vi "benchmark-DataContainer.vi"() -> (2 "read":dbl=1.454608345031738e-06 format="%#_6f", 3 "write":dbl=7.281229972839357e-07 format="%#_6f")   [LabVIEW 2017]
uses:
  0f9e4dc8-5c94-49e2-bb31-afcfc0247ef6.vi
  f88afbd5-defc-4e1d-9497-5b20b3cf386f.vi
  Data Container Folder/Support/Unflatten DataCNT to DVR.vi
  Data Container Folder/Data Container.lvlib
  <userlib>/_OpenG.lib/md5/md5.llb/MD5 Message Digest (Binary String)__ogtk.vi
panel:
  out "length":i32=1170
  out "outside":i32=499
  out "unit (ms)":cluster{dbl[]}[](graph)=[{[1.5038490295410156e-06, 1.503896713256836e-06, 1.4037609100341798e-06, 1.5039443969726562e-06, 1.503896713256836e-06, 1.4055252075195312e-06, 1.5020847320556641e-06, 1.5039920806884766e-06, 1.4037132263183594e-06, 1.503896713256836e-06, 1.4036178588867187e-06, 1.5039920806884766e-06, 1.503896713256836e-06, 1.4037132263183594e-06, 1.503896713256836e-06, 1.5039443969726562e-06, 1.4036655426025392e-06, 1.5039443969726562e-06, 1.4036655426025392e-06, 1.503896713256836e-06, 1.5039443969726562e-06, 1.40380859375e-06, 1.5038490295410156e-06, 1.4037132263183594e-06, 1.503896713256836e-06, 1.5039920806884766e-06, 1.4037132263183594e-06, 1.503896713256836e-06, 1.4036655426025392e-06, 1.4036178588867187e-06, 1.503896713256836e-06, 1.4037132263183594e-06, 1.503896713256836e-06, 1.4038562774658204e-06, 1.503753662109375e-06, 1.4036655426025392e-06, 1.4037609100341798e-06, 1.5039443969726562e-06, 1.503896713256836e-06, 1.5039443969726562e-06, 1.4036655426025392e-06, 1.5038490295410156e-06, 1.5039920806884766e-06, 1.5039443969726562e-06, 1.4037609100341798e-06, 1.503896713256836e-06, 1.5039443969726562e-06, 1.4036655426025392e-06, 1.503896713256836e-06, 1.6042709350585937e-06, 1.4035701751708983e-06, 1.4037132263183594e-06, 1.5039920806884766e-06, 1.503896713256836e-06, 1.4037132263183594e-06, 1.503896713256836e-06, 1.4036655426025392e-06, 1.4037132263183594e-06, 1.503896713256836e-06, 1.4036655426025392e-06, 1.5039443969726562e-06, 1.4036655426025392e-06, 1.4037132263183594e-06, 1.503896713256836e-06, 1.4036655426025392e-06, 1.5038490295410156e-06, 1.4037609100341798e-06, 1.4037609100341798e-06, 1.503896713256836e-06, 1.4036655426025392e-06, 1.5039443969726562e-06, 1.4036655426025392e-06, 1.5039920806884766e-06, 1.4036178588867187e-06, 1.4037609100341798e-06, 1.503896713256836e-06, 1.4036178588867187e-06, 1.4037609100341798e-06, 1.5039443969726562e-06, 1.4036655426025392e-06, 1.5039920806884766e-06, 1.4036178588867187e-06, 1.503896713256836e-06, 1.4036655426025392e-06, 1.4037132263183594e-06, 1.4036655426025392e-06, 1.5039443969726562e-06, 1.4035701751708983e-06, 1.5040874481201172e-06, 1.5039443969726562e-06, 1.4036655426025392e-06, 1.503896713256836e-06, 1.4037132263183594e-06, 1.503896713256836e-06, 1.4037132263183594e-06, 1.4035701751708983e-06, 1.5039920806884766e-06, 1.4037132263183594e-06, 1.503896713256836e-06, 1.4036655426025392e-06, 1.4037132263183594e-06, 1.503896713256836e-06, 1.4037132263183594e-06, 1.503896713256836e-06, 1.4036655426025392e-06, 1.4037132263183594e-06, 1.503896713256836e-06, 1.4036655426025392e-06, 1.5039443969726562e-06, 1.4036655426025392e-06, 1.4037132263183594e-06, 1.503896713256836e-06, 1.4036655426025392e-06, 1.604175567626953e-06, 1.4037609100341798e-06, 1.503896713256836e-06, 1.4037132263183594e-06, 1.5038490295410156e-06, 1.4037609100341798e-06, 1.5039920806884766e-06, 1.4035701751708983e-06, 1.4037132263183594e-06, 1.503896713256836e-06, 1.4036655426025392e-06, 1.5040397644042968e-06, 1.4035701751708983e-06, 1.4037132263183594e-06, 1.503896713256836e-06, 1.4036655426025392e-06, 1.4037132263183594e-06, 1.503896713256836e-06, 1.4036655426025392e-06, 1.4037132263183594e-06, 1.503896713256836e-06, 1.4036655426025392e-06, 1.4037132263183594e-06, 1.503896713256836e-06, 1.5039920806884766e-06, 1.4036178588867187e-06, 1.6042232513427735e-06, 1.5039443969726562e-06, 1.4036655426025392e-06, 1.4041900634765624e-06, 1.5034198760986327e-06, 1.4036655426025392e-06, 1.5039443969726562e-06, 1.4036655426025392e-06, 1.5039443969726562e-06, 1.4036655426025392e-06, 1.4036655426025392e-06, 1.8048286437988282e-06, 1.804637908935547e-06, 1.503896713256836e-06, 1.5039443969726562e-06, 1.5039920806884766e-06, 1.4036655426025392e-06, 1.5039443969726562e-06, 1.5039920806884766e-06, 1.4035701751708983e-06, 1.5039443969726562e-06, 1.4036655426025392e-06, 1.5039443969726562e-06, 1.4036655426025392e-06, 1.503896713256836e-06, 1.4037609100341798e-06, 1.5039443969726562e-06, 1.4036655426025392e-06, 1.5039443969726562e-06, 1.4035701751708983e-06, 1.4037132263183594e-06, 1.5039920806884766e-06, 1.4036655426025392e-06, 1.5039443969726562e-06, 1.4036655426025392e-06, 1.503896713256836e-06, 1.4037132263183594e-06, 1.503896713256836e-06, 1.4036655426025392e-06, 1.4037132263183594e-06, 1.503896713256836e-06, 1.4037132263183594e-06, 1.503896713256836e-06, 1.4036655426025392e-06, 1.5040397644042968e-06, 1.5038013458251954e-06, 1.4037132263183594e-06, 1.4036655426025392e-06, 1.5039920806884766e-06, 1.4036655426025392e-06, 1.4037132263183594e-06, 1.503896713256836e-06, 1.4037132263183594e-06, 1.503896713256836e-06, 1.4036655426025392e-06, 1.4037132263183594e-06, 1.503896713256836e-06, 1.4036655426025392e-06, 1.5039443969726562e-06, 1.4036655426025392e-06, 1.5039443969726562e-06, 1.4036655426025392e-06, 1.503896713256836e-06, 1.4037132263183594e-06, 1.503896713256836e-06, 1.4037609100341798e-06, 1.5038490295410156e-06, 1.4036655426025392e-06, 1.5040397644042968e-06, 1.4036655426025392e-06, 1.5038490295410156e-06, 1.4037609100341798e-06, 1.503896713256836e-06, 1.4036655426025392e-06, 1.5039443969726562e-06, 1.4036178588867187e-06, 1.4037132263183594e-06, 1.5039443969726562e-06, 1.4036655426025392e-06, 1.5039443969726562e-06, 1.503896713256836e-06, 1.4037132263183594e-06, 1.5039920806884766e-06, 1.4035701751708983e-06, 1.4037132263183594e-06, 1.5039920806884766e-06, 1.503896713256836e-06, 1.4036178588867187e-06, 1.5039920806884766e-06, 1.4036655426025392e-06, 1.5039443969726562e-06, 1.4036655426025392e-06, 1.4037132263183594e-06, 1.503896713256836e-06, 1.4036655426025392e-06, 1.5039443969726562e-06, 1.4036655426025392e-06, 1.5039443969726562e-06, 1.4036655426025392e-06, 1.503896713256836e-06, 1.4037132263183594e-06, 1.503896713256836e-06, 1.4036655426025392e-06, 1.5039443969726562e-06, 1.5039920806884766e-06, 1.4036655426025392e-06, 1.5038490295410156e-06, 1.4037609100341798e-06, 1.5039443969726562e-06, 1.4036655426025392e-06, 1.503896713256836e-06, 1.4037132263183594e-06, 1.503896713256836e-06, 1.4037132263183594e-06, 1.503896713256836e-06, 1.4036655426025392e-06, 1.5039443969726562e-06, 1.5039920806884766e-06, 1.4036655426025392e-06, 1.5039443969726562e-06, 1.4035701751708983e-06, 1.5040397644042968e-06, 1.4036655426025392e-06, 1.5038490295410156e-06, 1.4037609100341798e-06, 1.503896713256836e-06, 1.4037132263183594e-06, 1.503896713256836e-06, 1.4036655426025392e-06, 1.5039443969726562e-06, 1.4036655426025392e-06, 1.4036655426025392e-06, 1.5039443969726562e-06, 1.4036655426025392e-06, 1.5039443969726562e-06, 1.4036655426025392e-06, 1.5039920806884766e-06, 1.4036655426025392e-06, 1.5039443969726562e-06, 1.4036655426025392e-06, 1.5039443969726562e-06, 1.4036655426025392e-06, 1.5039443969726562e-06, 1.4036655426025392e-06, 1.4036655426025392e-06, 1.5039443969726562e-06, 1.4036655426025392e-06, 1.503896713256836e-06, 1.4037132263183594e-06, 1.503896713256836e-06, 1.4036655426025392e-06, 1.5039443969726562e-06, 1.4036655426025392e-06, 1.5039443969726562e-06, 1.4036655426025392e-06, 1.5039920806884766e-06, 1.4037132263183594e-06, 1.5038013458251954e-06, 1.4037132263183594e-06, 1.5039920806884766e-06, 1.4036655426025392e-06, 1.5039443969726562e-06, 1.503896713256836e-06, 1.4036655426025392e-06, 1.5039443969726562e-06, 1.4036655426025392e-06, 1.4037132263183594e-06, 1.503896713256836e-06, 1.4036655426025392e-06, 1.5039920806884766e-06, 1.5038490295410156e-06, 1.4037132263183594e-06, 1.4036655426025392e-06, 1.503896713256836e-06, 1.5040397644042968e-06, 1.4036655426025392e-06, 1.4035701751708983e-06, 1.5040397644042968e-06, 1.4036655426025392e-06, 1.503896713256836e-06, 1.5039443969726562e-06, 1.4036655426025392e-06, 1.5039443969726562e-06, 1.4036655426025392e-06, 1.503896713256836e-06, 1.5039443969726562e-06, 1.4037609100341798e-06, 1.503896713256836e-06, 1.5039443969726562e-06, 1.503896713256836e-06, 1.4037132263183594e-06, 1.503896713256836e-06, 1.4037132263183594e-06, 1.4035701751708983e-06, 1.5039920806884766e-06, 1.5039443969726562e-06, 1.4036655426025392e-06, 1.4036655426025392e-06, 1.5039443969726562e-06, 1.4036655426025392e-06, 1.5039443969726562e-06, 1.4036655426025392e-06, 1.5039920806884766e-06, 1.4036655426025392e-06, 1.5039443969726562e-06, 1.4036655426025392e-06, 1.5039443969726562e-06, 1.4036655426025392e-06, 1.5039443969726562e-06, 1.4036655426025392e-06, 1.503896713256836e-06, 1.4037132263183594e-06, 1.4036655426025392e-06, 1.503896713256836e-06, 1.5039443969726562e-06, 1.4037609100341798e-06, 1.503896713256836e-06, 1.4035224914550781e-06, 1.5040874481201172e-06, 1.4036178588867187e-06, 1.5039920806884766e-06, 1.4036178588867187e-06, 1.503896713256836e-06, 1.4041423797607422e-06, 1.5035629272460938e-06, 1.4036655426025392e-06, 1.503896713256836e-06, 1.4037132263183594e-06, 1.503896713256836e-06, 1.4036655426025392e-06, 1.5039443969726562e-06, 1.5039920806884766e-06, 1.4036655426025392e-06, 1.4036178588867187e-06, 1.5039920806884766e-06, 1.4036178588867187e-06, 1.4036655426025392e-06, 1.5039443969726562e-06, 1.4037609100341798e-06, 1.503896713256836e-06, 1.4036655426025392e-06, 1.5039443969726562e-06, 1.503896713256836e-06, 1.4037132263183594e-06, 1.5039920806884766e-06, 1.4035701751708983e-06, 1.5039443969726562e-06, 1.4037609100341798e-06, 1.4036178588867187e-06, 1.503896713256836e-06, 1.4036655426025392e-06, 1.5039443969726562e-06, 1.4036655426025392e-06, 1.5039920806884766e-06, 1.4036178588867187e-06, 1.5039920806884766e-06, 1.4036655426025392e-06, 1.5050411224365234e-06, 1.4025688171386718e-06, 1.604175567626953e-06, 1.4037609100341798e-06, 1.4035701751708983e-06, 1.5039443969726562e-06, 1.4036655426025392e-06, 1.5039443969726562e-06, 1.4036655426025392e-06, 1.5039443969726562e-06, 1.4036655426025392e-06, 1.503896713256836e-06, 1.4037609100341798e-06, 1.4036178588867187e-06, 1.503896713256836e-06, 1.4037132263183594e-06, 1.503896713256836e-06, 1.4037609100341798e-06, 1.5038490295410156e-06, 1.4036655426025392e-06, 1.5039443969726562e-06, 1.40380859375e-06, 1.5038490295410156e-06, 1.4037132263183594e-06, 1.503896713256836e-06, 1.4036655426025392e-06, 1.4037132263183594e-06, 1.503896713256836e-06, 1.4036655426025392e-06, 1.5039443969726562e-06, 1.4036655426025392e-06, 1.5039443969726562e-06, 1.4036655426025392e-06, 1.4036655426025392e-06, 1.5039920806884766e-06, 1.4036178588867187e-06, 1.5039443969726562e-06, 1.4036655426025392e-06, 1.5039920806884766e-06, 1.4036655426025392e-06, 1.4037132263183594e-06, 1.503896713256836e-06, 1.4036178588867187e-06, 1.5039920806884766e-06, 1.4036655426025392e-06, 1.5039443969726562e-06, 1.4036655426025392e-06, 1.4036655426025392e-06, 1.5039443969726562e-06, 1.4036655426025392e-06, 1.5039443969726562e-06, 1.4036655426025392e-06, 1.4036655426025392e-06, 1.5039443969726562e-06, 1.4036655426025392e-06, 1.5039443969726562e-06, 1.4036655426025392e-06, 1.5039920806884766e-06, 1.4036178588867187e-06, 1.4036655426025392e-06, 1.503896713256836e-06, 1.4037132263183594e-06, 1.503896713256836e-06, 1.4037132263183594e-06, 1.4036655426025392e-06, 1.5039920806884766e-06, 1.4036178588867187e-06, 1.5039920806884766e-06, 1.4035701751708983e-06, 1.4037132263183594e-06, 1.5039920806884766e-06, 1.5038490295410156e-06, 1.4037609100341798e-06, 1.503896713256836e-06, 1.4038562774658204e-06, 1.4035224914550781e-06, 1.503896713256836e-06, 1.4037132263183594e-06, 1.503896713256836e-06, 1.4037609100341798e-06, 1.4036178588867187e-06, 1.503896713256836e-06, 1.4036178588867187e-06, 1.5039920806884766e-06, 1.4037609100341798e-06, 1.5038490295410156e-06, 1.4037609100341798e-06, 1.5038013458251954e-06, 1.4037132263183594e-06, 1.503896713256836e-06, 1.5039920806884766e-06, 1.4037132263183594e-06, 1.503896713256836e-06, 1.5039443969726562e-06, 1.503896713256836e-06, 1.4037609100341798e-06, 1.4037132263183594e-06, 1.5038013458251954e-06, 1.4037132263183594e-06, 1.503896713256836e-06, 1.4037609100341798e-06, 1.5039443969726562e-06, 1.4036655426025392e-06, 1.4043331146240235e-06]}, ...(2 in all)]
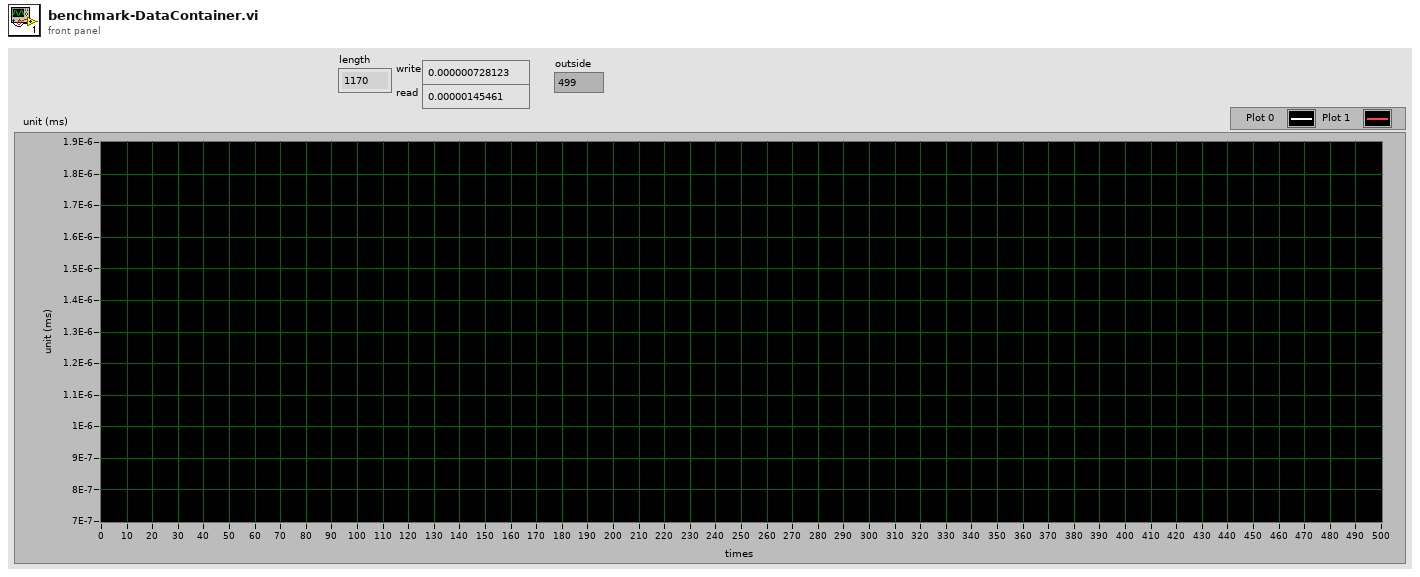
[diagram p1: front panel]
types:
  T1 = cluster{"error constant":errorcluster, "error constant 2":errorcluster, "error constant 3":errorcluster, "error constant 4":errorcluster, "error constant 5":errorcluster, "error constant 6":errorcluster, "error constant 7":errorcluster, "error constant 8":errorcluster, "error constant 9":errorcluster, "error constant 10":errorcluster, "error constant 11":errorcluster, "error constant 12":errorcluster, "error constant 13":errorcluster, "error constant 14":errorcluster, "error constant 15":errorcluster, "error constant 16":errorcluster, "error constant 17":errorcluster, "error constant 18":errorcluster, "error constant 19":errorcluster, "error constant 20":errorcluster, "error constant 21":errorcluster, "error constant 22":errorcluster, "error constant 23":errorcluster, "error constant 24":errorcluster, "error constant 25":errorcluster, "error constant 26":errorcluster, "error constant 27":errorcluster, "error constant 28":errorcluster, "error constant 29":errorcluster, "error constant 30":errorcluster, "error constant 31":errorcluster, "error constant 32":errorcluster, "error constant 33":errorcluster, "error constant 34":errorcluster, "error constant 35":errorcluster, "error constant 36":errorcluster, "error constant 37":errorcluster, "error constant 38":errorcluster, "error constant 39":errorcluster, "error constant 40":errorcluster, "error constant 41":errorcluster, "error constant 42":errorcluster, "error constant 43":errorcluster, "error constant 44":errorcluster, "error constant 45":errorcluster, "error constant 46":errorcluster, "error constant 47":errorcluster, "error constant 48":errorcluster, "error constant 49":errorcluster, "error constant 50":errorcluster, "error constant 51":errorcluster, "error constant 52":errorcluster, "error constant 53":errorcluster, "error constant 54":errorcluster, "error constant 55":errorcluster, "error constant 56":errorcluster, "error constant 57":errorcluster, "error constant 58":errorcluster, "error constant 59":errorcluster, "error constant 60":errorcluster, "error constant 61":errorcluster, "error constant 62":errorcluster, "error constant 63":errorcluster, "error constant 64":errorcluster, "error constant 65":errorcluster, cluster{"error constant":errorcluster, "error constant 2":errorcluster, "error constant 3":errorcluster, "error constant 4":errorcluster, "error constant 5":errorcluster, "error constant 6":errorcluster, "error constant 7":errorcluster, "error constant 8":errorcluster, "error constant 9":errorcluster, "error constant 10":errorcluster, "error constant 11":errorcluster, "error constant 12":errorcluster, "error constant 13":errorcluster, "error constant 14":errorcluster, "error constant 15":errorcluster, "error constant 16":errorcluster, "error constant 17":errorcluster, "error constant 18":errorcluster, "error constant 19":errorcluster, "error constant 20":errorcluster, "error constant 21":errorcluster, "error constant 22":errorcluster, "error constant 23":errorcluster, "error constant 24":errorcluster, "error constant 25":errorcluster, "error constant 26":errorcluster, "error constant 27":errorcluster, "error constant 28":errorcluster, "error constant 29":errorcluster, "error constant 30":errorcluster, "error constant 31":errorcluster, "error constant 32":errorcluster, "error constant 33":errorcluster, "error constant 34":errorcluster, "error constant 35":errorcluster, "error constant 36":errorcluster, "error constant 37":errorcluster, "error constant 38":errorcluster, "error constant 39":errorcluster, "error constant 40":errorcluster, "error constant 41":errorcluster, "error constant 42":errorcluster, "error constant 43":errorcluster, "error constant 44":errorcluster, "error constant 45":errorcluster, "error constant 46":errorcluster, "error constant 47":errorcluster, "error constant 48":errorcluster, "error constant 49":errorcluster, "error constant 50":errorcluster, "error constant 51":errorcluster, "error constant 52":errorcluster, "error constant 53":errorcluster, "error constant 54":errorcluster, "error constant 55":errorcluster, "error constant 56":errorcluster, "error constant 57":errorcluster, "error constant 58":errorcluster, "error constant 59":errorcluster, "error constant 60":errorcluster, "error constant 61":errorcluster, "error constant 62":errorcluster, "error constant 63":errorcluster, "error constant 64":errorcluster, "error constant 65":errorcluster}}
  T2 = typedef "Data Container.lvlib/Def-DataCNT.ctl" = refnum<k1>
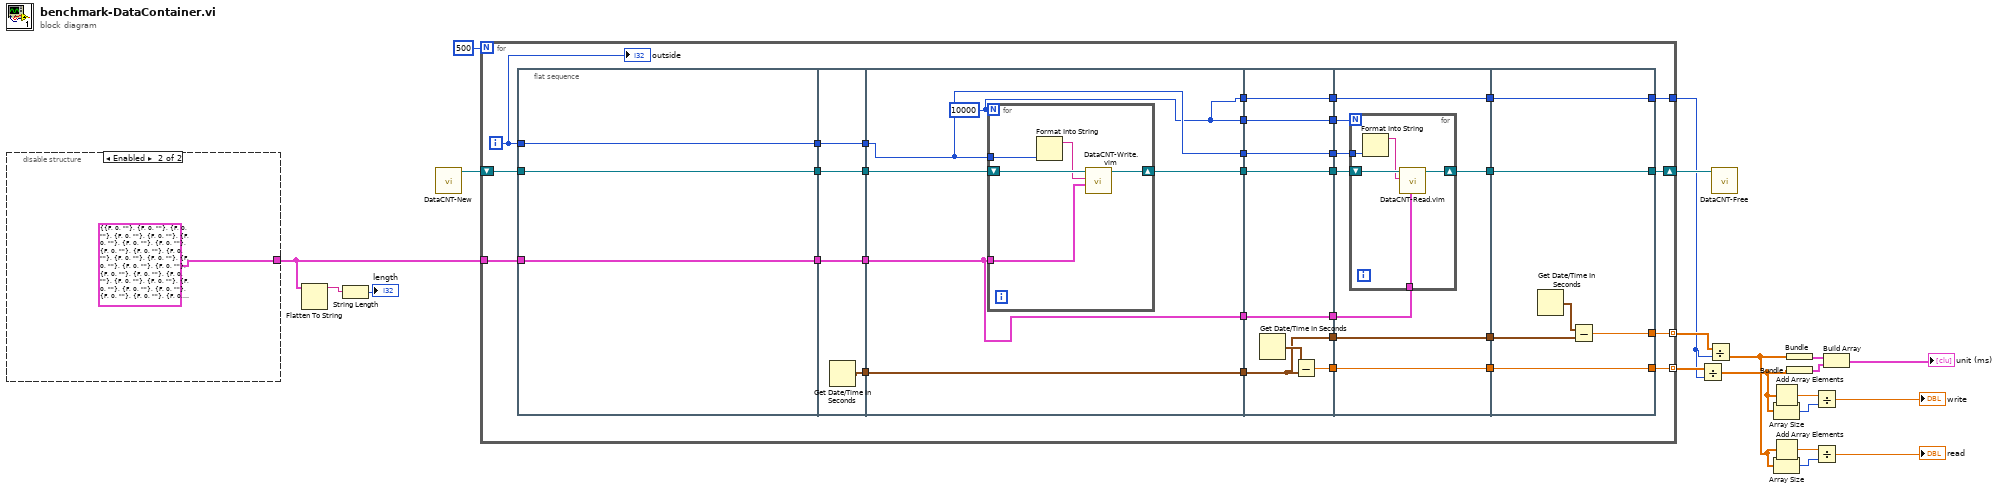
[diagram p0: block diagram]
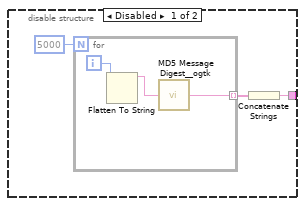
[diagram p2: hidden frame]
diagram:
  n1 = disable-structure shown="Enabled" {
    disable-tunnel: [w21 T1 {"error constant"={"status"=FALSE, "code"=0, "source"=""}, "error constant 2"={"status"=FALSE, "code"=0, "source"=""}, "error constant 3"={"status"=FALSE, "code"=0, "source"=""}, "error constant 4"={"status"=FALSE, "code"=0, "source"=""}, "error constant 5"={"status"=FALSE, "code"=0, "source"=""}, "error constant 6"={"status"=FALSE, "code"=0, "source"=""}, "error constant 7"={"status"=FALSE, "code"=0, "source"=""}, "error constant 8"={"status"=FALSE, "code"=0, "source"=""}, "error constant 9"={"status"=FALSE, "code"=0, "source"=""}, "error constant 10"={"status"=FALSE, "code"=0, "source"=""}, "error constant 11"={"status"=FALSE, "code"=0, "source"=""}, "error constant 12"={"status"=FALSE, "code"=0, "source"=""}, "error constant 13"={"status"=FALSE, "code"=0, "source"=""}, "error constant 14"={"status"=FALSE, "code"=0, "source"=""}, "error constant 15"={"status"=FALSE, "code"=0, "source"=""}, "error constant 16"={"status"=FALSE, "code"=0, "source"=""}, "error constant 17"={"status"=FALSE, "code"=0, "source"=""}, "error constant 18"={"status"=FALSE, "code"=0, "source"=""}, "error constant 19"={"status"=FALSE, "code"=0, "source"=""}, "error constant 20"={"status"=FALSE, "code"=0, "source"=""}, "error constant 21"={"status"=FALSE, "code"=0, "source"=""}, "error constant 22"={"status"=FALSE, "code"=0, "source"=""}, "error constant 23"={"status"=FALSE, "code"=0, "source"=""}, "error constant 24"={"status"=FALSE, "code"=0, "source"=""}, "error constant 25"={"status"=FALSE, "code"=0, "source"=""}, "error constant 26"={"status"=FALSE, "code"=0, "source"=""}, "error constant 27"={"status"=FALSE, "code"=0, "source"=""}, "error constant 28"={"status"=FALSE, "code"=0, "source"=""}, "error constant 29"={"status"=FALSE, "code"=0, "source"=""}, "error constant 30"={"status"=FALSE, "code"=0, "source"=""}, "error constant 31"={"status"=FALSE, "code"=0, "source"=""}, "error constant 32"={"status"=FALSE, "code"=0, "source"=""}, "error constant 33"={"status"=FALSE, "code"=0, "source"=""}, "error constant 34"={"status"=FALSE, "code"=0, "source"=""}, "error constant 35"={"status"=FALSE, "code"=0, "source"=""}, "error constant 36"={"status"=FALSE, "code"=0, "source"=""}, "error constant 37"={"status"=FALSE, "code"=0, "source"=""}, "error constant 38"={"status"=FALSE, "code"=0, "source"=""}, "error constant 39"={"status"=FALSE, "code"=0, "source"=""}, "error constant 40"={"status"=FALSE, "code"=0, "source"=""}, "error constant 41"={"status"=FALSE, "code"=0, "source"=""}, "error constant 42"={"status"=FALSE, "code"=0, "source"=""}, "error constant 43"={"status"=FALSE, "code"=0, "source"=""}, "error constant 44"={"status"=FALSE, "code"=0, "source"=""}, "error constant 45"={"status"=FALSE, "code"=0, "source"=""}, "error constant 46"={"status"=FALSE, "code"=0, "source"=""}, "error constant 47"={"status"=FALSE, "code"=0, "source"=""}, "error constant 48"={"status"=FALSE, "code"=0, "source"=""}, "error constant 49"={"status"=FALSE, "code"=0, "source"=""}, "error constant 50"={"status"=FALSE, "code"=0, "source"=""}, "error constant 51"={"status"=FALSE, "code"=0, "source"=""}, "error constant 52"={"status"=FALSE, "code"=0, "source"=""}, "error constant 53"={"status"=FALSE, "code"=0, "source"=""}, "error constant 54"={"status"=FALSE, "code"=0, "source"=""}, "error constant 55"={"status"=FALSE, "code"=0, "source"=""}, "error constant 56"={"status"=FALSE, "code"=0, "source"=""}, "error constant 57"={"status"=FALSE, "code"=0, "source"=""}, "error constant 58"={"status"=FALSE, "code"=0, "source"=""}, "error constant 59"={"status"=FALSE, "code"=0, "source"=""}, "error constant 60"={"status"=FALSE, "code"=0, "source"=""}, "error constant 61"={"status"=FALSE, "code"=0, "source"=""}, "error constant 62"={"status"=FALSE, "code"=0, "source"=""}, "error constant 63"={"status"=FALSE, "code"=0, "source"=""}, "error constant 64"={"status"=FALSE, "code"=0, "source"=""}, "error constant 65"={"status"=FALSE, "code"=0, "source"=""}, {"error constant"={"status"=FALSE, "code"=0, "source"=""}, "error constant 2"={"status"=FALSE, "code"=0, "source"=""}, "error constant 3"={"status"=FALSE, "code"=0, "source"=""}, "error constant 4"={"status"=FALSE, "code"=0, "source"=""}, "error constant 5"={"status"=FALSE, "code"=0, "source"=""}, "error constant 6"={"status"=FALSE, "code"=0, "source"=""}, "error constant 7"={"status"=FALSE, "code"=0, "source"=""}, "error constant 8"={"status"=FALSE, "code"=0, "source"=""}, "error constant 9"={"status"=FALSE, "code"=0, "source"=""}, "error constant 10"={"status"=FALSE, "code"=0, "source"=""}, "error constant 11"={"status"=FALSE, "code"=0, "source"=""}, "error constant 12"={"status"=FALSE, "code"=0, "source"=""}, "error constant 13"={"status"=FALSE, "code"=0, "source"=""}, "error constant 14"={"status"=FALSE, "code"=0, "source"=""}, "error constant 15"={"status"=FALSE, "code"=0, "source"=""}, "error constant 16"={"status"=FALSE, "code"=0, "source"=""}, "error constant 17"={"status"=FALSE, "code"=0, "source"=""}, "error constant 18"={"status"=FALSE, "code"=0, "source"=""}, "error constant 19"={"status"=FALSE, "code"=0, "source"=""}, "error constant 20"={"status"=FALSE, "code"=0, "source"=""}, "error constant 21"={"status"=FALSE, "code"=0, "source"=""}, "error constant 22"={"status"=FALSE, "code"=0, "source"=""}, "error constant 23"={"status"=FALSE, "code"=0, "source"=""}, "error constant 24"={"status"=FALSE, "code"=0, "source"=""}, "error constant 25"={"status"=FALSE, "code"=0, "source"=""}, "error constant 26"={"status"=FALSE, "code"=0, "source"=""}, "error constant 27"={"status"=FALSE, "code"=0, "source"=""}, "error constant 28"={"status"=FALSE, "code"=0, "source"=""}, "error constant 29"={"status"=FALSE, "code"=0, "source"=""}, "error constant 30"={"status"=FALSE, "code"=0, "source"=""}, "error constant 31"={"status"=FALSE, "code"=0, "source"=""}, "error constant 32"={"status"=FALSE, "code"=0, "source"=""}, "error constant 33"={"status"=FALSE, "code"=0, "source"=""}, "error constant 34"={"status"=FALSE, "code"=0, "source"=""}, "error constant 35"={"status"=FALSE, "code"=0, "source"=""}, "error constant 36"={"status"=FALSE, "code"=0, "source"=""}, "error constant 37"={"status"=FALSE, "code"=0, "source"=""}, "error constant 38"={"status"=FALSE, "code"=0, "source"=""}, "error constant 39"={"status"=FALSE, "code"=0, "source"=""}, "error constant 40"={"status"=FALSE, "code"=0, "source"=""}, "error constant 41"={"status"=FALSE, "code"=0, "source"=""}, "error constant 42"={"status"=FALSE, "code"=0, "source"=""}, "error constant 43"={"status"=FALSE, "code"=0, "source"=""}, "error constant 44"={"status"=FALSE, "code"=0, "source"=""}, "error constant 45"={"status"=FALSE, "code"=0, "source"=""}, "error constant 46"={"status"=FALSE, "code"=0, "source"=""}, "error constant 47"={"status"=FALSE, "code"=0, "source"=""}, "error constant 48"={"status"=FALSE, "code"=0, "source"=""}, "error constant 49"={"status"=FALSE, "code"=0, "source"=""}, "error constant 50"={"status"=FALSE, "code"=0, "source"=""}, "error constant 51"={"status"=FALSE, "code"=0, "source"=""}, "error constant 52"={"status"=FALSE, "code"=0, "source"=""}, "error constant 53"={"status"=FALSE, "code"=0, "source"=""}, "error constant 54"={"status"=FALSE, "code"=0, "source"=""}, "error constant 55"={"status"=FALSE, "code"=0, "source"=""}, "error constant 56"={"status"=FALSE, "code"=0, "source"=""}, "error constant 57"={"status"=FALSE, "code"=0, "source"=""}, "error constant 58"={"status"=FALSE, "code"=0, "source"=""}, "error constant 59"={"status"=FALSE, "code"=0, "source"=""}, "error constant 60"={"status"=FALSE, "code"=0, "source"=""}, "error constant 61"={"status"=FALSE, "code"=0, "source"=""}, "error constant 62"={"status"=FALSE, "code"=0, "source"=""}, "error constant 63"={"status"=FALSE, "code"=0, "source"=""}, "error constant 64"={"status"=FALSE, "code"=0, "source"=""}, "error constant 65"={"status"=FALSE, "code"=0, "source"=""}}}] -> w15
    frame Disabled {
      n2 = for {
        N: 5000 -> [_]
        tunnel: [w26] -> w23 mode=indexing
        i -> [w25]
        n3 = Flatten To String(anything=w25) -> (data string=w24:string)  [unwired: 3 in, 2 out]
        n4 = call-poly <userlib>:"MD5 Message Digest__ogtk.vi"("Message"=w24) -> ("MD5 Message Digest"=w26:string)
      }
      n5 = Concatenate Strings(w23) -> (w21:string)
    }
    frame Enabled {
    }
  }
  n6 = Flatten To String(anything=w15) -> (data string=w14:string)  [unwired: 3 in, 2 out]
  n7 = String Length(string=w14) -> (length=→"length":i32)
  n8 = call "DataCNT-New.vi"() -> ("DataCNT out"=w17:T2)  [unwired: 10 in, 1 out]
  n9 = for {
    N: 500 -> [_]
    tunnel: [w56] -> w20 mode=indexing
    tunnel: [w55] -> w1
    tunnel: w15 -> [w42]
    shift-right: [w40] -> w16
    shift-left: w17 -> [w41]
    tunnel: [w35] -> w2 mode=indexing
    i -> [w53]
    n10 = flat-sequence {
      tunnel: w53 -> [w61]
      tunnel: [w59] -> w47
      tunnel: [w60] -> w45
      tunnel: [w61] -> w44
      tunnel: w42 -> [w60]
      tunnel: w41 -> [w59]
      tunnel: [w65] -> w58
      tunnel: [w64] -> w48
      tunnel: w47 -> [w64]
      tunnel: [w63] -> w46
      tunnel: w45 -> [w63]
      tunnel: w44 -> [w62]
      tunnel: [w62] -> w43
      tunnel: w58 -> [w71]
      tunnel: [w71] -> w57
      tunnel: [w67] -> w54
      tunnel: [w69] -> w49
      tunnel: w48 -> [w70]
      tunnel: w46 -> [w66]
      tunnel: w43 -> [w68]
      tunnel: [w67] -> w33
      tunnel: [w68] -> w30
      tunnel: [w66] -> w29
      tunnel: w57 -> [w80]
      tunnel: w54 -> [w82]
      tunnel: [w83] -> w52
      tunnel: [w82] -> w51
      tunnel: [w81] -> w50
      tunnel: w49 -> [w81]
      tunnel: [w80] -> w37
      tunnel: w33 -> [w79]
      tunnel: [w79] -> w32
      tunnel: [w78] -> w31
      tunnel: w30 -> [w78]
      tunnel: w29 -> [w77]
      tunnel: [w77] -> w28
      tunnel: w52 -> [w92]
      tunnel: w51 -> [w91]
      tunnel: w50 -> [w89]
      tunnel: [w92] -> w39
      tunnel: [w91] -> w38
      tunnel: w37 -> [w90]
      tunnel: [w90] -> w36
      tunnel: [w88] -> w34
      tunnel: w32 -> [w87]
      tunnel: w31 -> [w86]
      tunnel: w28 -> [w85]
      tunnel: [w101] -> w40
      tunnel: [w102] -> w55
      tunnel: [w103] -> w56
      tunnel: w39 -> [w103]
      tunnel: w38 -> [w102]
      tunnel: w36 -> [w99]
      tunnel: [w98] -> w35
      tunnel: w34 -> [w101]
      frame #0 {
      }
      frame #1 {
        n11 = Get Date/Time In Seconds() -> (seconds since 1Jan1904=w65:timestamp)
      }
      frame #2 {
        w67 = 10000
        n12 = for {
          N: w67 -> [_]
          tunnel: w66 -> [w74]
          tunnel: w68 -> [w73]
          shift-right: [w75] -> w69
          shift-left: w70 -> [w76]
          n13 = Format Into String(w73) -> (resulting string=w72:string)  [unwired: 3 in, 1 out]
          n14 = call "DataCNT-Write.vim"("Value"=w74, "Name"=w72, "DataCNT"=w76) -> ("DataCNT(dup)"=w75:T2)  [unwired: 5 in, 3 out]
        }
      }
      frame #3 {
        n15 = Get Date/Time In Seconds() -> (seconds since 1Jan1904=w84:timestamp)
        n16 = Subtract(x=w84, y=w80) -> (x-y=w83:dbl)
      }
      frame #4 {
        n17 = for {
          N: w87 -> [_]
          shift-right: [w96] -> w88
          shift-left: w89 -> [w97]
          tunnel: w86 -> [w94]
          tunnel: w85 -> [w93]
          n18 = Format Into String(w94) -> (resulting string=w95:string)  [unwired: 3 in, 1 out]
          n19 = call "DataCNT-Read.vim"("Type"=w93, "Name"=w95, "DataCNT"=w97) -> ("DataCNT(dup)"=w96:T2)  [unwired: 4 in, 4 out]
        }
      }
      frame #5 {
        n20 = Get Date/Time In Seconds() -> (seconds since 1Jan1904=w100:timestamp)
        n21 = Subtract(x=w100, y=w99) -> (x-y=w98:dbl)
      }
    }
    "outside" <- w53
  }
  n22 = Divide(x=w20, y=w1) -> (x/y=w10:dbl[])
  n23 = Divide(x=w2, y=w1) -> (x/y=w3:dbl[])
  n24 = call "DataCNT-Free.vi"("DataCNT"=w16) -> ()  [unwired: 10 in, 1 out]
  n25 = Add Array Elements(numeric array=w10) -> (sum=w12:dbl)
  n26 = Array Size(array=w10) -> (size(s)=w11:i32)
  n27 = Add Array Elements(numeric array=w3) -> (sum=w5:dbl)
  n28 = Array Size(array=w3) -> (size(s)=w6:i32)
  n29 = Bundle(w3) -> (w9:cluster{dbl[]})  [unwired: 1 in]
  n30 = Bundle(w10) -> (w8:cluster{dbl[]})  [unwired: 1 in]
  n31 = Divide(x=w12, y=w11) -> (x/y=→"write":dbl)
  n32 = Divide(x=w5, y=w6) -> (x/y=→"read":dbl)
  n33 = Build Array(w9, w8) -> (→"unit (ms)":cluster{dbl[]}[])
